vi "Test Sequencer.vi"(0 "WaitingData":bool, 1 "TestRunning?":bool, 2 "Stabilized?":bool, 3 "Stabilized":refnum<vi>, 5 "StepDataActive":dbl format="%#_13g", 7 "FreeFlow":bool, 9 "StepTimeLimit":dbl format="%#_13g", 11 "State Array In":string[](array[string]), 12 "LastDataTime":i64, 13 "StableCount":dbl format="%#_13g", 14 "TestType":enum32{"Flow", "Test", "Hot\nFuel"}(ring)) -> (4 "FreezeCmdPID":bool, 15 "State Array Out":string[](array[string]))   [LabVIEW 2019]
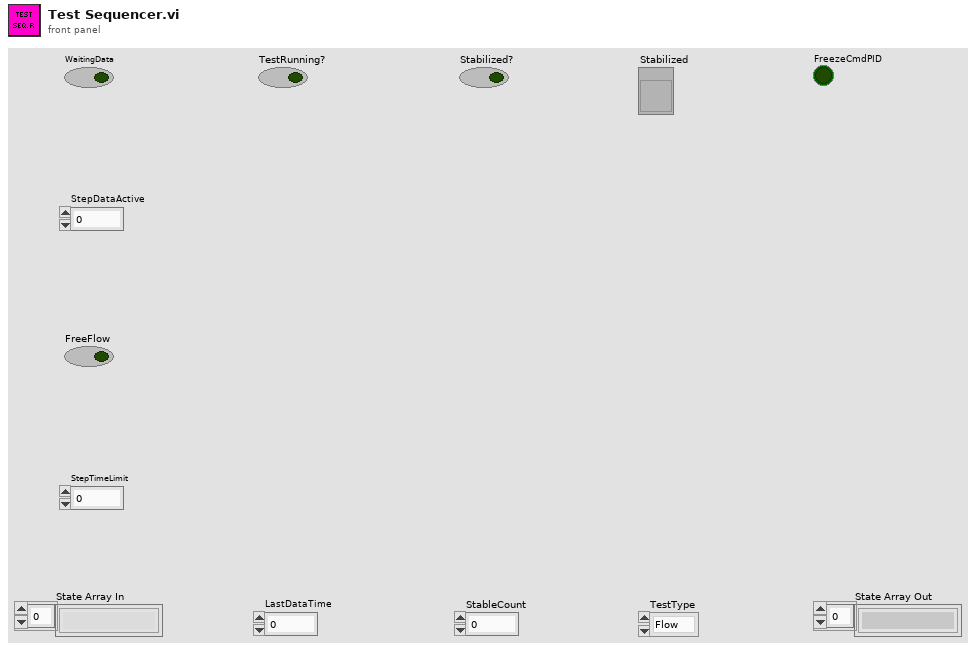
[diagram p1: front panel]
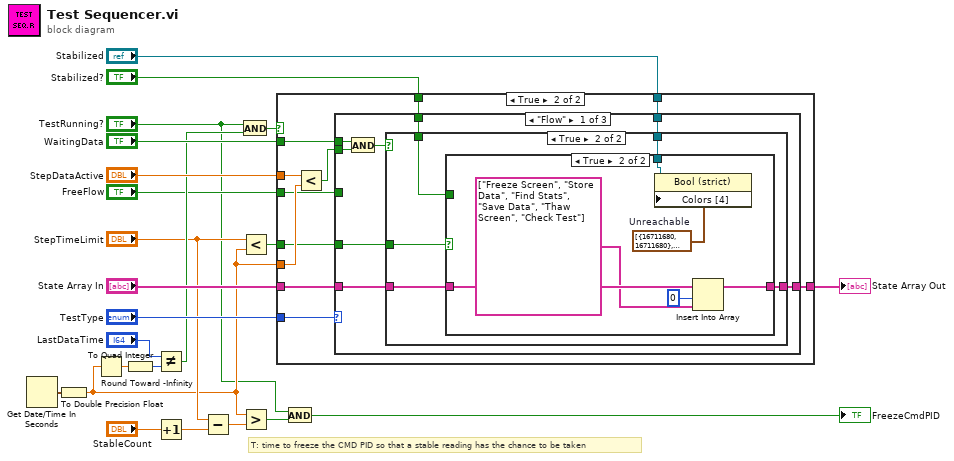
[diagram p0: block diagram]
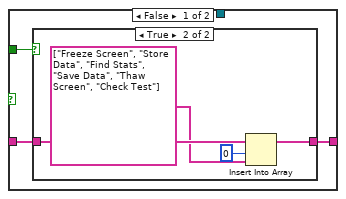
[diagram p4: hidden frame]
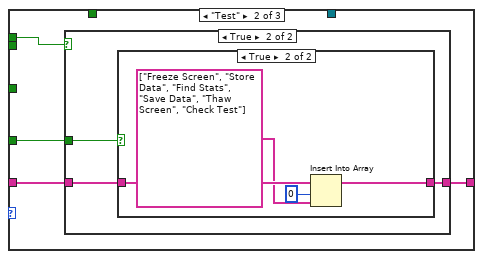
[diagram p6: hidden frame]
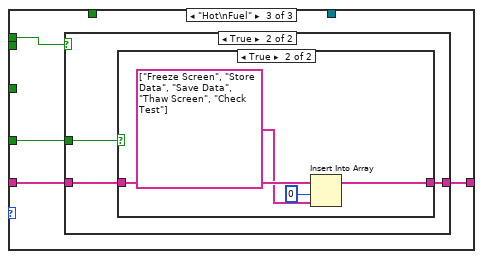
[diagram p9: hidden frame]
diagram:
  # "T: time to freeze the CMD PID so that a stable reading has the chance to be taken"
  n1 = Get Date/Time In Seconds() -> (seconds since 1Jan1904=w15:timestamp)
  n2 = To Double Precision Float(number=w15) -> (double precision float=w6:dbl)
  n3 = Round Toward -Infinity(1:w6) -> (0:w16:dbl)
  n4 = To Quad Integer(1:w16) -> (0:w1:i64)
  n5 = Not Equal?(x="LastDataTime", y=w1) -> (x != y?=w13:bool)
  n6 = Increment(x="StableCount") -> (x+1=w7:dbl)
  n7 = Subtract(x="StepTimeLimit", y=w7) -> (x-y=w5:dbl)
  n8 = And(x="TestRunning?", y=w13) -> (x .and. y?=w17:bool)
  n9 = Less?(x="StepTimeLimit", y=w6) -> (x < y?=w11:bool)
  n10 = Greater?(x=w6, y=w5) -> (0:w4:bool)
  n11 = case shown="True" w17 {
    tunnel: "WaitingData" -> [_ w28]
    tunnel: w6 -> [_ w30]
    tunnel: "State Array In" -> [w24 w34]
    tunnel: "Stabilized?" -> [_ w32]
    tunnel: "TestType" -> [_ w35]
    tunnel: [w24 w33] -> w22
    tunnel: "StepDataActive" -> [_ w31]
    tunnel: "FreeFlow" -> [_ w29]
    tunnel: w11 -> [_ w26]
    tunnel: "Stabilized" -> [_ w25]
    frame False {
    }
    frame True {
      n12 = Less?(x=w31, y=w30) -> (x < y?=w27:bool)
      n13 = case shown="\"Flow\"" w35 {
        tunnel: w34 -> [w43 w67 w80]
        tunnel: [w42 w66 w79] -> w33
        tunnel: w32 -> [w41 _ _]
        tunnel: w29 -> [_ _ _]
        tunnel: w28 -> [w40 w64 w78]
        tunnel: w27 -> [w39 _ _]
        tunnel: w26 -> [w38 w65 w77]
        tunnel: w25 -> [w36 _ _]
        frame "Flow" {
          n14 = And(x=w40, y=w39) -> (x .and. y?=w37:bool)
          n15 = case shown="True" w37 {
            tunnel: w43 -> [w44 w48]
            tunnel: [w44 w47] -> w42
            tunnel: w41 -> [_ w49]
            tunnel: w38 -> [_ w46]
            tunnel: w36 -> [_ w45]
            frame False {
            }
            frame True {
              n16 = case shown="True" w46 {
                tunnel: w49 -> [w51 _]
                tunnel: w48 -> [w52 w61]
                tunnel: [w50 w59] -> w47
                tunnel: w45 -> [_ w58]
                frame False {
                  n17 = case shown="True" w51 {
                    tunnel: w52 -> [w53 w56]
                    tunnel: [w53 w54] -> w50
                    frame False {
                    }
                    frame True {
                      n18 = Insert Into Array(array=w56, index=0, new element=string[] ["Freeze Screen", "Store Data", "Find Stats", "Save Data", "Thaw Screen", "Check Test"]) -> (w54:string[])
                    }
                  }
                }
                frame True {
                  w63 = cluster{u32, u32}[] [{16711680, 16711680}, {8978432, 8978432}, {8323072, 8323072}, {4456448, 4456448}]  # Unreachable
                  n19 = property on="Property Node" class="Bool (strict)"(reference=w58, "Colors [4]"=w63) -> ()  [unwired: 1 in, 2 out]
                  n20 = Insert Into Array(array=w61, index=0, new element=string[] ["Freeze Screen", "Store Data", "Find Stats", "Save Data", "Thaw Screen", "Check Test"]) -> (w59:string[])
                }
              }
            }
          }
        }
        frame "Test" {
          n21 = case shown="True" w64 {
            tunnel: w67 -> [w68 w71]
            tunnel: [w68 w70] -> w66
            tunnel: w65 -> [_ w69]
            frame False {
            }
            frame True {
              n22 = case shown="True" w69 {
                tunnel: w71 -> [w72 w75]
                tunnel: [w72 w73] -> w70
                frame False {
                }
                frame True {
                  n23 = Insert Into Array(array=w75, index=0, new element=string[] ["Freeze Screen", "Store Data", "Find Stats", "Save Data", "Thaw Screen", "Check Test"]) -> (w73:string[])
                }
              }
            }
          }
        }
        frame "Hot\nFuel" {
          n24 = case shown="True" w78 {
            tunnel: w80 -> [w81 w84]
            tunnel: [w81 w83] -> w79
            tunnel: w77 -> [_ w82]
            frame False {
            }
            frame True {
              n25 = case shown="True" w82 {
                tunnel: w84 -> [w85 w88]
                tunnel: [w85 w86] -> w83
                frame False {
                }
                frame True {
                  n26 = Insert Into Array(array=w88, index=0, new element=string[] ["Freeze Screen", "Store Data", "Save Data", "Thaw Screen", "Check Test"]) -> (w86:string[])
                }
              }
            }
          }
        }
      }
    }
  }
  "State Array Out" <- w22
  n27 = And(x="TestRunning?", y=w4) -> (x .and. y?=→"FreezeCmdPID":bool)
